vi "time.vi"(9 "new value (time)":dbl, 11 "buffer in (time)":dbl[](array[numeric])) -> (0 "dt":dbl, 1 "-delta t":dbl, 3 "buffer out (time)":dbl[](array[numeric]))   [LabVIEW 2010, in "Licor-Steuerung.lvlib"]
uses:
  Licor-Steuerung.lvlib
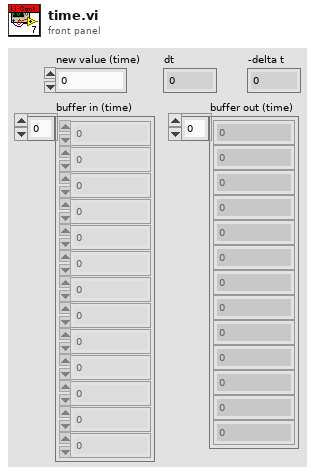
[diagram p1: front panel]
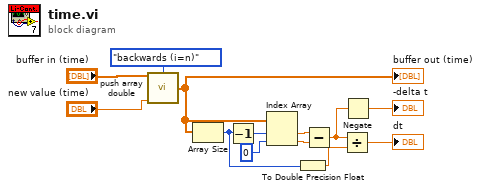
[diagram p0: block diagram]
diagram:
  n1 = call "push array double.vi"("Array"="buffer in (time)", "mode"=enum16{"forwards (i=0)", "backwards (i=n)"}."backwards (i=n)", "Element"="new value (time)") -> ("Array out"=w3:dbl[])  [unwired: 12 in]
  "buffer out (time)" <- w3
  n2 = Array Size(array=w3) -> (size(s)=w5:i32)
  n3 = Decrement(x=w5) -> (x-1=w11:i32)
  n4 = Index Array(array=w3, index #1=w11, index #2=0 ("Index")) -> (element #1=w12:dbl, element #2=w13:dbl)
  n5 = To Double Precision Float(number=w5) -> (double precision float=w6:dbl)
  n6 = Subtract(x=w12, y=w13) -> (x-y=w8:dbl)
  n7 = Divide(x=w8, y=w6) -> (x/y=→"dt":dbl)
  n8 = Negate(x=w8) -> (-x=→"-delta t":dbl)
